vi "Read Authenticated.vi"(8 "Error In":errorcluster, 11 "Session In":refnum<class "Session.lvclass">) -> (0 "Error Out":errorcluster, 2 "Authenticated":bool, 3 "Sesssion Out":refnum<class "Session.lvclass">)   [LabVIEW 2018, in "Toolkit.lvlib" / "Session.lvclass"]
uses:
  Session.lvclass
  Session.lvclass/Session.ctl
  SSH/SSH.lvclass/SSH.ctl
  Toolkit.lvlib
  SSH/SSH.lvclass
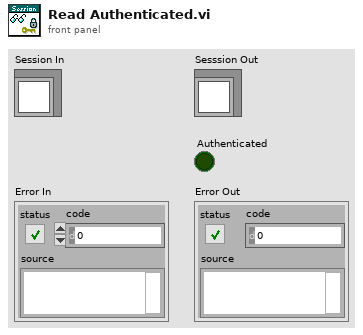
[diagram p1: front panel]
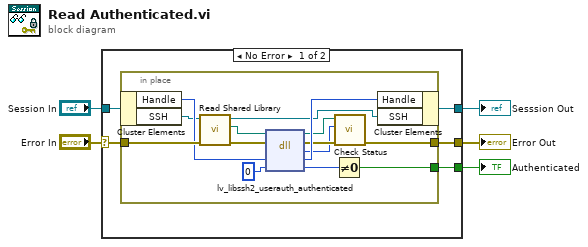
[diagram p0: block diagram]
diagram:
  n1 = case shown="No Error" "Error In" {
    selector: "Error In" -> [w9 w26]
    tunnel: [w10 w26] -> w4
    tunnel: "Session In" -> [w8 w25]
    tunnel: [w7 w25] -> w2
    tunnel: [w6 _] -> w1
    frame No Error {
      n2 = in-place {
        in-place-border: [w20] -> w10
        in-place-border: w9 -> [w24]
        in-place-border: [w15] -> w6
        n3 = in-place-cluster #1(w8) -> ("Handle"=w23:u64, "SSH"=w13:refnum<class "SSH.lvclass">)
        n4 = call "Read Shared Library.vi"("Error In"=w24, "SSH In"=w13) -> ("Error Out"=w14:errorcluster, "lv-libssh2 Shared Library"=w12:path, "SSH Out"=w11:refnum<class "SSH.lvclass">)  [unwired: 7 in]
        n5 = dll-call lib="D:/Users/cfield/Code/Field R&D Services/SSH/LV-LIBSSH2/LabVIEW/trunk/src/Toolkit/Support/lv-libssh2.*" fn="lv_libssh2_userauth_authenticated"(path in=w12, error in=w14, "session"=w23, "authenticated"=0 ("mode")) -> (path out=w19:path, error out=w21:errorcluster, "status"=w18:i32, "session"=w22:u64, "authenticated"=w16:i32)  [unwired: 1 in]
        n6 = Not Equal To 0?(x=w16) -> (x != 0?=w15:bool)
        n7 = call "Check Status.vi"("Error In"=w21, "Status"=w18, "lv-libssh2 Shared Library In"=w19) -> ("Error Out"=w20:errorcluster)  [unwired: 7 in, 1 out]
        n8 = in-place-cluster #1("Handle"=w22, "SSH"=w11) -> (w7:refnum<class "Session.lvclass">)
      }
    }
    frame Error {
    }
  }
  "Sesssion Out" <- w2
  "Error Out" <- w4
  "Authenticated" <- w1
